vi "409b_main.vi"(0 "Synth":T1(array[cluster])=[{"AC Frequency (kHz)"=0.0, " Initial AC Ampl. (p-p/2)"=0.4, "Final AC Ampl."=0.4, "Frequency(MHz)"=0.0, "Phase(rad)"=0.0, "Voltage(%)"=0.0, "Gamma AC"=1.0, "String"="Channel 0 A", "Blanck"=0.0}, {"AC Frequency (kHz)"=0.0, " Initial AC Ampl. (p-p/2)"=0.4, "Final AC Ampl."=0.4, "Frequency(MHz)"=0.0, "Phase(rad)"=0.0, "Voltage(%)"=0.0, "Gamma AC"=1.0, "String"="Channel 0 B", "Blanck"=0.0}, {"AC Frequency (kHz)"=0.0, " Initial AC Ampl. (p-p/2)"=0.4, "Final AC Ampl."=0.4, "Frequency(MHz)"=75.0, "Phase(rad)"=0.0, "Voltage(%)"=100.0, "Gamma AC"=1.0, "String"="Channel 0 C", "Blanck"=0.0}, {"AC Frequency (kHz)"=0.0, " Initial AC Ampl. (p-p/2)"=0.4, "Final AC Ampl."=0.4, "Frequency(MHz)"=146.3, "Phase(rad)"=0.0, "Voltage(%)"=100.0, "Gamma AC"=1.0, "String"="Channel 0 D", "Blanck"=0.0}, {"AC Frequency (kHz)"=0.0, " Initial AC Ampl. (p-p/2)"=0.0, "Final AC Ampl."=0.0, "Frequency(MHz)"=0.6, "Phase(rad)"=1.0, "Voltage(%)"=1.0, "Gamma AC"=0.0, "String"="Channel 0 E", "Blanck"=0.2}] {"Blanck" format="%.2f"; "Gamma AC" format="%.2f"; "Voltage(%)" min=0.0 max=100.0 step=1.0; "Phase(rad)" min=0.0 max=6.383118 format="%#_4f"; "Frequency(MHz)" min=0.0 max=150.0 format="%.7f"; "Final AC Ampl." format="%.3f"; "Initial AC Ampl. (p-p/2)" format="%.3f"; "AC Frequency (kHz)" format="%.2f"}, 1 "cmd":string, 2 "?":bool, 3 "Turn Table Mode On When Run?\n(Stays in table mode if already in it.) The default setup should be \"Set Frequency Manually\" and \"X\".":bool=TRUE, 4 "Set Channel 0":bool, 5 "Set Channel 1":bool, 6 "Set Channel 2":bool, 7 "Set Channel 3":bool, 8 "Port":refnum<visa-resource-name>="COM5") -> ()   [LabVIEW 2013]
uses:
  Instance           2 17Saved   409b_main .vi
  Instance           4 17Saved   409b_main .vi
  Instance           5 17Saved   409b_main .vi
  Instance           6 17Saved   409b_main .vi
  Instance           7 17Saved   409b_main .vi
panel:
  out "rp3":string
  out "rf3":string
  out "rv3":string
  out "rp2":string
  out "rf2":string
  out "rv2":string
  out "rp1":string
  out "rf1":string
  out "rv1":string
  out "rv0":string
  out "Results":string[][](table)=[["d1 0000\r\n357EC360,0000,03FF,FF OK\r\n", "1", "0000", "89.750000", "0", "100", "FF"], ["d0 0000\r\n357EC360,0000,03FF,FF OK\r\n", "0", "0000", "89.750000", "0", "100", "FF"], ["d1 0001\r\n35CB0EA0,0000,03FF,00 OK\r\n", "1", "0001", "90.250000", "0", "100", "00"], ["d0 0001\r\n35CB0EA0,0000,03FF,00 OK\r\n", "0", "0001", "90.250000", "0", "100", "00"]] caption="results"
  in  "Table":string[][](table)=[["1", "0000", "89.75", "0", "100", "ff"], ["0", "0000", "89.75", "0", "100", "ff"], ["1", "0001", "90.25", "0", "100", "00"], ["0", "0001", "90.25", "0", "100", "00"], ["", "", "", "", "", ""], ["", "", "", "", "", ""]] caption="Commands 90 MHz for 88Sr; 73.82 MHz for 86Sr"
  out "rcmd0":string="\r\nOK\r\n"
  out "rf0":string
  out "rp0":string
  # "Set Frequency Manually/ Table Mode"
  # "(If in table mode, setting channel 0 and 1 does nothing.)"
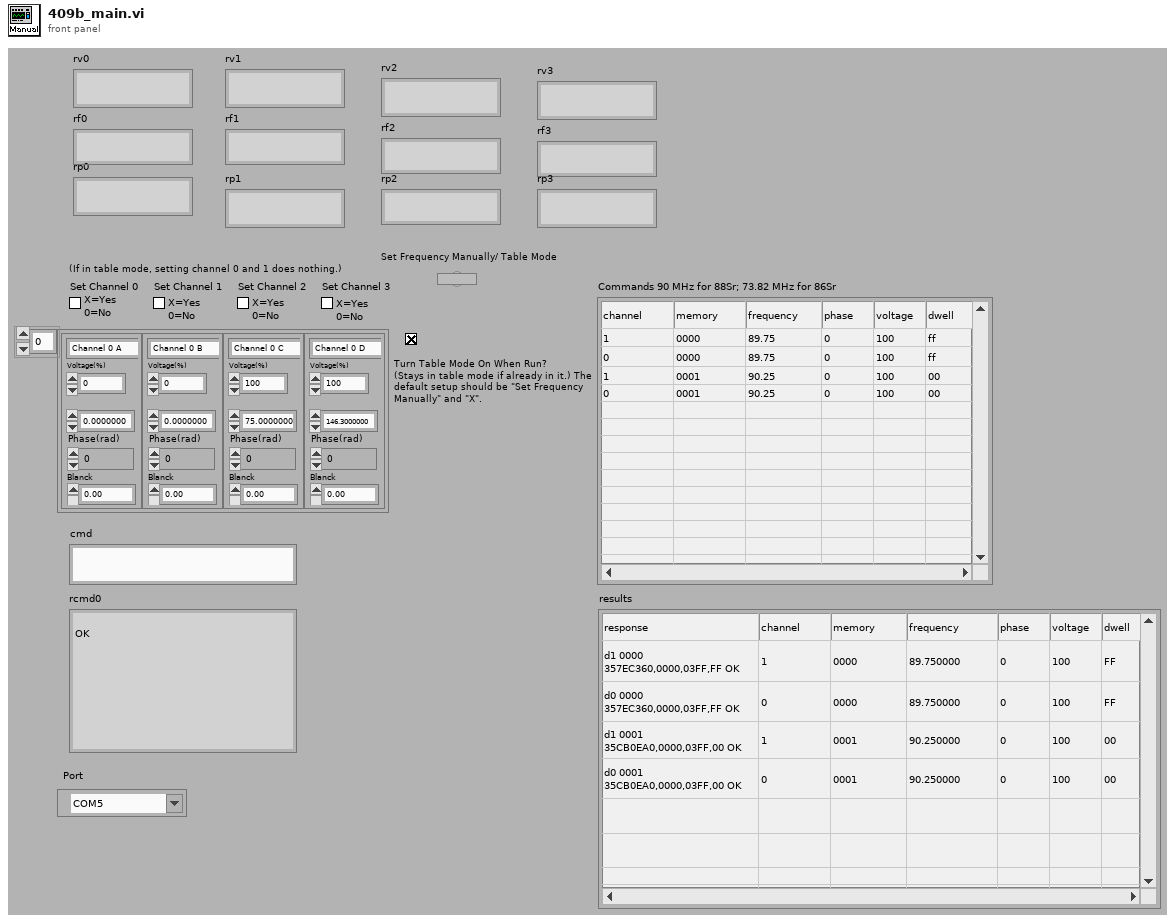
[diagram p1: front panel]
types:
  T1 = cluster{"AC Frequency (kHz)":dbl, " Initial AC Ampl. (p-p/2)":dbl, "Final AC Ampl.":dbl, "Frequency(MHz)":dbl, "Phase(rad)":dbl, "Voltage(%)":dbl, "Gamma AC":dbl, "String":string, "Blanck":dbl}[]
  T2 = cluster{"AC Frequency (kHz)":dbl, " Initial AC Ampl. (p-p/2)":dbl, "Final AC Ampl.":dbl, "Frequency(MHz)":dbl, "Phase(rad)":dbl, "Voltage(%)":dbl, "Gamma AC":dbl, "String":string, "Blanck":dbl}
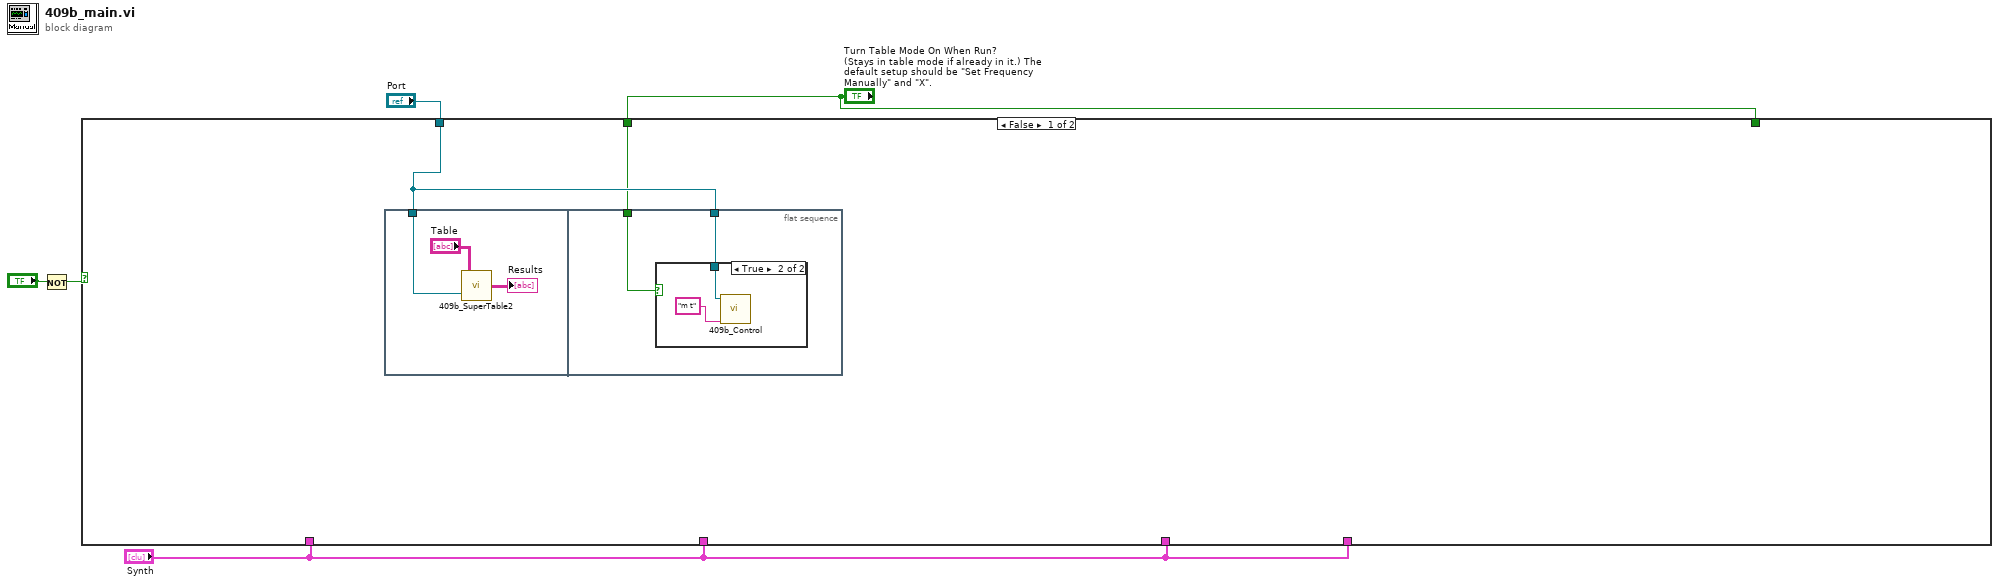
[diagram p0: block diagram]
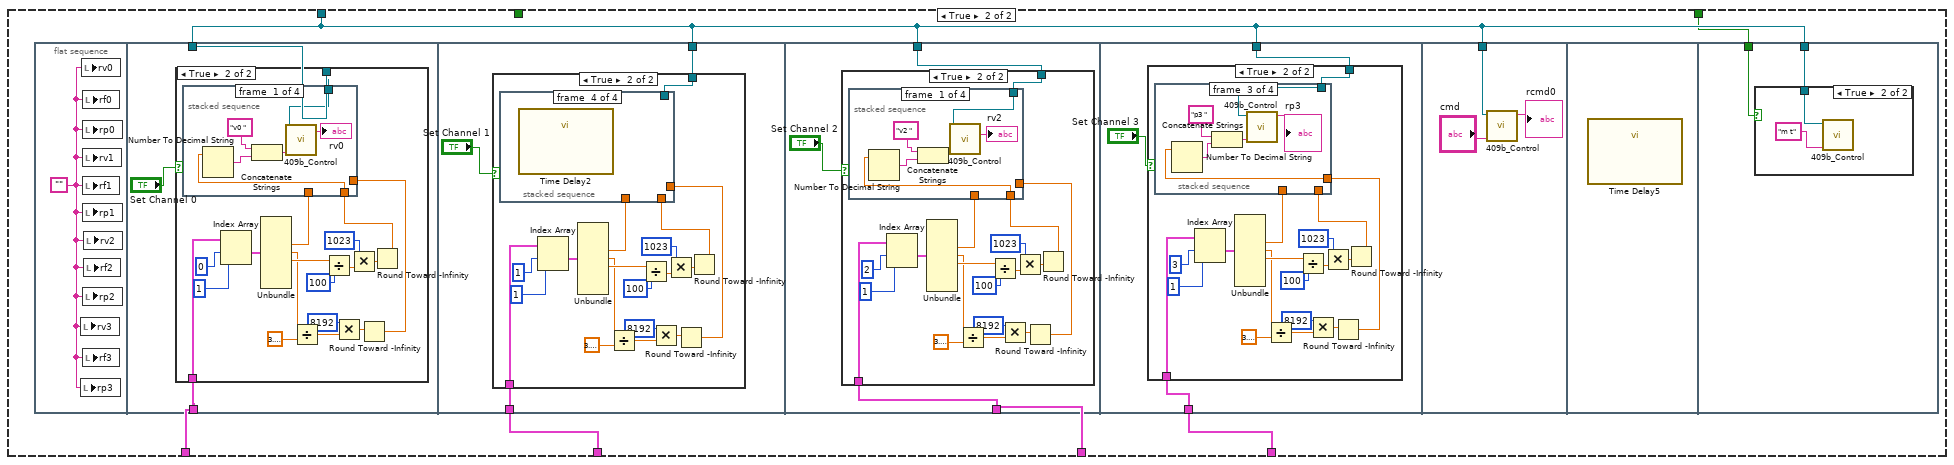
[diagram p3: hidden frame]
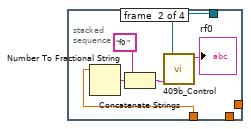
[diagram p5: hidden frame]
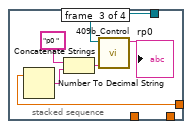
[diagram p6: hidden frame]
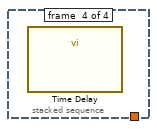
[diagram p7: hidden frame]
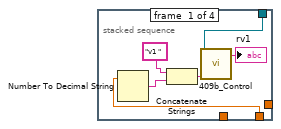
[diagram p9: hidden frame]
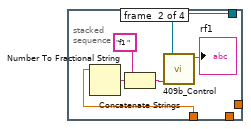
[diagram p10: hidden frame]
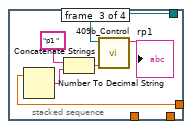
[diagram p11: hidden frame]
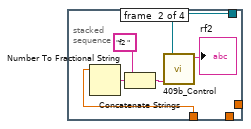
[diagram p13: hidden frame]
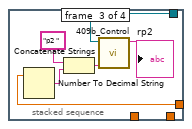
[diagram p14: hidden frame]
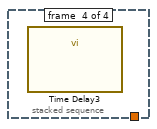
[diagram p15: hidden frame]
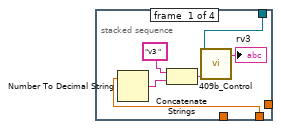
[diagram p17: hidden frame]
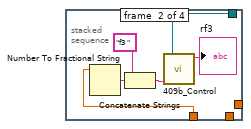
[diagram p18: hidden frame]
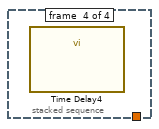
[diagram p19: hidden frame]
diagram:
  n1 = Not(x="?") -> (.not. x?=w2:bool)
  n2 = case shown="False" w2 {
    tunnel: "Port" -> [w7 w16]
    tunnel: "Synth" -> [_ w20]
    tunnel: "Synth" -> [_ w19]
    tunnel: "Synth" -> [_ w18]
    tunnel: "Synth" -> [_ w17]
    tunnel: "Turn Table Mode On When Run?\n(Stays in table mode if already in it.) The default setup should be \"Set Frequency Manually\" and \"X\"." -> [w6 _]
    tunnel: "Turn Table Mode On When Run?\n(Stays in table mode if already in it.) The default setup should be \"Set Frequency Manually\" and \"X\"." -> [_ w15]
    frame False {
      n3 = flat-sequence {
        tunnel: w7 -> [w8]
        tunnel: w7 -> [w12]
        tunnel: w6 -> [w11]
        frame #0 {
          n4 = call "409b_SuperTable2.vi"("Port"=w8, "Table"="Table") -> ("Results2"=→"Results":string[][])
        }
        frame #1 {
          n5 = case shown="True" w11 {
            tunnel: w12 -> [_ w13]
            frame False {
            }
            frame True {
              n6 = call "409b_Control.vi"("Port"=w13, "Command"="m t") -> ()  [unwired: 8 in, 1 out]
            }
          }
        }
      }
    }
    frame True {
      n7 = flat-sequence {
        tunnel: w16 -> [w24]
        tunnel: w20 -> [w22]
        tunnel: w16 -> [w61]
        tunnel: w19 -> [w63]
        tunnel: w16 -> [w101]
        tunnel: w18 -> [w100]
        tunnel: w16 -> [w140]
        tunnel: w17 -> [w139]
        tunnel: w16 -> [w178]
        tunnel: w16 -> [w182]
        tunnel: w15 -> [w181]
        frame #0 {
          w21 = ""
          n8 = local write "rv3"(w21) -> ()
          n9 = local write "rp3"(w21) -> ()
          n10 = local write "rv0"(w21) -> ()
          n11 = local write "rf0"(w21) -> ()
          n12 = local write "rp0"(w21) -> ()
          n13 = local write "rv1"(w21) -> ()
          n14 = local write "rf1"(w21) -> ()
          n15 = local write "rp1"(w21) -> ()
          n16 = local write "rp2"(w21) -> ()
          n17 = local write "rf3"(w21) -> ()
          n18 = local write "rv2"(w21) -> ()
          n19 = local write "rf2"(w21) -> ()
        }
        frame #1 {
          n20 = case shown="True" "Set Channel 0" {
            tunnel: w24 -> [_ w42]
            tunnel: w22 -> [_ w39]
            frame False {
            }
            frame True {
              n21 = Index Array(array=w39, index #1=0, index #2=1) -> (element #1=w38:T2)  [unwired: 1 out]
              n22 = Unbundle(w38) -> ("Frequency(MHz)"=w37:dbl, "Phase(rad)"=w27:dbl, "Voltage(%)"=w36:dbl)  [unwired: 6 out]
              n23 = Divide(x=w27, y=3.141592653589793) -> (x/y=w30:dbl)
              n24 = Divide(x=w36, y=100) -> (x/y=w35:dbl)
              n25 = Multiply(x=8192, y=w30) -> (x*y=w28:dbl)
              n26 = Multiply(x=1023, y=w35) -> (x*y=w33:dbl)
              n27 = Round Toward -Infinity(1:w28) -> (0:w25:dbl)
              n28 = Round Toward -Infinity(1:w33) -> (0:w32:dbl)
              n29 = stacked-sequence {
                tunnel: w42 -> [w46 w52 w57 _]
                tunnel: w37 -> [_ w50 _ _]
                tunnel: w32 -> [w44 _ _ _]
                tunnel: w25 -> [_ _ w55 _]
                frame #0 {
                  n30 = Number To Decimal String(number=w44) -> (decimal integer string=w45:string)  [unwired: 1 in]
                  n31 = Concatenate Strings("v0 ", w45) -> (w47:string)
                  n32 = call "409b_Control.vi"("Port"=w46, "Command"=w47) -> ("Response"=→"rv0":string)  [unwired: 8 in]
                }
                frame #1 {
                  n33 = Number To Fractional String(number=w50) -> (F-format string=w49:string)  [unwired: 3 in]
                  n34 = Concatenate Strings("f0 ", w49) -> (w54:string)
                  n35 = call "409b_Control.vi"("Port"=w52, "Command"=w54) -> ("Response"=→"rf0":string)  [unwired: 8 in]
                }
                frame #2 {
                  n36 = Number To Decimal String(number=w55) -> (decimal integer string=w56:string)  [unwired: 1 in]
                  n37 = Concatenate Strings("p0 ", w56) -> (w59:string)
                  n38 = call "409b_Control.vi"("Port"=w57, "Command"=w59) -> ("Response"=→"rp0":string)  [unwired: 8 in]
                }
                frame #3 {
                  n39 = call "Time Delay"() -> ()  [unwired: 11 in, 1 out]
                }
              }
            }
          }
        }
        frame #2 {
          n40 = case shown="True" "Set Channel 1" {
            tunnel: w63 -> [_ w79]
            tunnel: w61 -> [_ w64]
            frame False {
            }
            frame True {
              n41 = Index Array(array=w79, index #1=1, index #2=1) -> (element #1=w78:T2)  [unwired: 1 out]
              n42 = Unbundle(w78) -> ("Frequency(MHz)"=w77:dbl, "Phase(rad)"=w67:dbl, "Voltage(%)"=w76:dbl)  [unwired: 6 out]
              n43 = Divide(x=w67, y=3.141592653589793) -> (x/y=w70:dbl)
              n44 = Divide(x=w76, y=100) -> (x/y=w75:dbl)
              n45 = Multiply(x=8192, y=w70) -> (x*y=w68:dbl)
              n46 = Multiply(x=1023, y=w75) -> (x*y=w73:dbl)
              n47 = Round Toward -Infinity(1:w68) -> (0:w65:dbl)
              n48 = Round Toward -Infinity(1:w73) -> (0:w72:dbl)
              n49 = stacked-sequence {
                tunnel: w64 -> [w85 w91 w96 _]
                tunnel: w77 -> [_ w89 _ _]
                tunnel: w72 -> [w83 _ _ _]
                tunnel: w65 -> [_ _ w94 _]
                frame #0 {
                  n50 = Number To Decimal String(number=w83) -> (decimal integer string=w84:string)  [unwired: 1 in]
                  n51 = Concatenate Strings("v1 ", w84) -> (w86:string)
                  n52 = call "409b_Control.vi"("Port"=w85, "Command"=w86) -> ("Response"=→"rv1":string)  [unwired: 8 in]
                }
                frame #1 {
                  n53 = Number To Fractional String(number=w89) -> (F-format string=w88:string)  [unwired: 3 in]
                  n54 = Concatenate Strings("f1 ", w88) -> (w93:string)
                  n55 = call "409b_Control.vi"("Port"=w91, "Command"=w93) -> ("Response"=→"rf1":string)  [unwired: 8 in]
                }
                frame #2 {
                  n56 = Number To Decimal String(number=w94) -> (decimal integer string=w95:string)  [unwired: 1 in]
                  n57 = Concatenate Strings("p1 ", w95) -> (w98:string)
                  n58 = call "409b_Control.vi"("Port"=w96, "Command"=w98) -> ("Response"=→"rp1":string)  [unwired: 8 in]
                }
                frame #3 {
                  n59 = call "Time Delay2"() -> ()  [unwired: 11 in, 1 out]
                }
              }
            }
          }
        }
        frame #3 {
          n60 = case shown="True" "Set Channel 2" {
            tunnel: w100 -> [_ w118]
            tunnel: w101 -> [_ w103]
            frame False {
            }
            frame True {
              n61 = Index Array(array=w118, index #1=2, index #2=1) -> (element #1=w117:T2)  [unwired: 1 out]
              n62 = Unbundle(w117) -> ("Frequency(MHz)"=w116:dbl, "Phase(rad)"=w106:dbl, "Voltage(%)"=w115:dbl)  [unwired: 6 out]
              n63 = Divide(x=w106, y=3.141592653589793) -> (x/y=w109:dbl)
              n64 = Divide(x=w115, y=100) -> (x/y=w114:dbl)
              n65 = Multiply(x=8192, y=w109) -> (x*y=w107:dbl)
              n66 = Multiply(x=1023, y=w114) -> (x*y=w112:dbl)
              n67 = Round Toward -Infinity(1:w107) -> (0:w104:dbl)
              n68 = Round Toward -Infinity(1:w112) -> (0:w111:dbl)
              n69 = stacked-sequence {
                tunnel: w103 -> [w124 w130 w135 _]
                tunnel: w116 -> [_ w128 _ _]
                tunnel: w111 -> [w122 _ _ _]
                tunnel: w104 -> [_ _ w133 _]
                frame #0 {
                  n70 = Number To Decimal String(number=w122) -> (decimal integer string=w123:string)  [unwired: 1 in]
                  n71 = Concatenate Strings("v2 ", w123) -> (w125:string)
                  n72 = call "409b_Control.vi"("Port"=w124, "Command"=w125) -> ("Response"=→"rv2":string)  [unwired: 8 in]
                }
                frame #1 {
                  n73 = Number To Fractional String(number=w128) -> (F-format string=w127:string)  [unwired: 3 in]
                  n74 = Concatenate Strings("f2 ", w127) -> (w132:string)
                  n75 = call "409b_Control.vi"("Port"=w130, "Command"=w132) -> ("Response"=→"rf2":string)  [unwired: 8 in]
                }
                frame #2 {
                  n76 = Number To Decimal String(number=w133) -> (decimal integer string=w134:string)  [unwired: 1 in]
                  n77 = Concatenate Strings("p2 ", w134) -> (w137:string)
                  n78 = call "409b_Control.vi"("Port"=w135, "Command"=w137) -> ("Response"=→"rp2":string)  [unwired: 8 in]
                }
                frame #3 {
                  n79 = call "Time Delay3"() -> ()  [unwired: 11 in, 1 out]
                }
              }
            }
          }
        }
        frame #4 {
          n80 = case shown="True" "Set Channel 3" {
            tunnel: w139 -> [_ w157]
            tunnel: w140 -> [_ w142]
            frame False {
            }
            frame True {
              n81 = Index Array(array=w157, index #1=3, index #2=1) -> (element #1=w156:T2)  [unwired: 1 out]
              n82 = Unbundle(w156) -> ("Frequency(MHz)"=w155:dbl, "Phase(rad)"=w145:dbl, "Voltage(%)"=w154:dbl)  [unwired: 6 out]
              n83 = Divide(x=w145, y=3.141592653589793) -> (x/y=w148:dbl)
              n84 = Divide(x=w154, y=100) -> (x/y=w153:dbl)
              n85 = Multiply(x=8192, y=w148) -> (x*y=w146:dbl)
              n86 = Multiply(x=1023, y=w153) -> (x*y=w151:dbl)
              n87 = Round Toward -Infinity(1:w146) -> (0:w143:dbl)
              n88 = Round Toward -Infinity(1:w151) -> (0:w150:dbl)
              n89 = stacked-sequence {
                tunnel: w142 -> [w163 w169 w174 _]
                tunnel: w155 -> [_ w167 _ _]
                tunnel: w150 -> [w161 _ _ _]
                tunnel: w143 -> [_ _ w172 _]
                frame #0 {
                  n90 = Number To Decimal String(number=w161) -> (decimal integer string=w162:string)  [unwired: 1 in]
                  n91 = Concatenate Strings("v3 ", w162) -> (w164:string)
                  n92 = call "409b_Control.vi"("Port"=w163, "Command"=w164) -> ("Response"=→"rv3":string)  [unwired: 8 in]
                }
                frame #1 {
                  n93 = Number To Fractional String(number=w167) -> (F-format string=w166:string)  [unwired: 3 in]
                  n94 = Concatenate Strings("f3 ", w166) -> (w171:string)
                  n95 = call "409b_Control.vi"("Port"=w169, "Command"=w171) -> ("Response"=→"rf3":string)  [unwired: 8 in]
                }
                frame #2 {
                  n96 = Number To Decimal String(number=w172) -> (decimal integer string=w173:string)  [unwired: 1 in]
                  n97 = Concatenate Strings("p3 ", w173) -> (w176:string)
                  n98 = call "409b_Control.vi"("Port"=w174, "Command"=w176) -> ("Response"=→"rp3":string)  [unwired: 8 in]
                }
                frame #3 {
                  n99 = call "Time Delay4"() -> ()  [unwired: 11 in, 1 out]
                }
              }
            }
          }
        }
        frame #5 {
          n100 = call "409b_Control.vi"("Port"=w178, "Command"="cmd") -> ("Response"=→"rcmd0":string)  [unwired: 8 in]
        }
        frame #6 {
          n101 = call "Time Delay5"() -> ()  [unwired: 11 in, 1 out]
        }
        frame #7 {
          n102 = case shown="True" w181 {
            tunnel: w182 -> [_ w183]
            frame False {
            }
            frame True {
              n103 = call "409b_Control.vi"("Port"=w183, "Command"="m t") -> ()  [unwired: 8 in, 1 out]
            }
          }
        }
      }
    }
  }
